vi "Read RequestMessage.vi"(8 "error in (no error)":errorcluster, 11 "HttpResponseMessage in":refnum<class "HttpResponseMessage.lvclass">) -> (0 "error out":errorcluster, 2 "HttpRequestMessage out":refnum<class "HttpRequestMessage.lvclass">, 3 "HttpResponseMessage out":refnum<class "HttpResponseMessage.lvclass">)   [LabVIEW 2018, in "LabVIEWHTTPClient_NET.lvlib" / "HttpResponseMessage.lvclass"]
uses:
  HttpResponseMessage.lvclass
  HttpRequestMessage/HttpRequestMessage.lvclass
  HttpResponseMessage.lvclass/HttpResponseMessage.ctl
  System.Net.Http
  Accessors/Write HttpRequestMessage.vi
  Accessors/Read NET_HttpReponseMessage.vi
  Accessors/Read HttpRequestMessage.vi
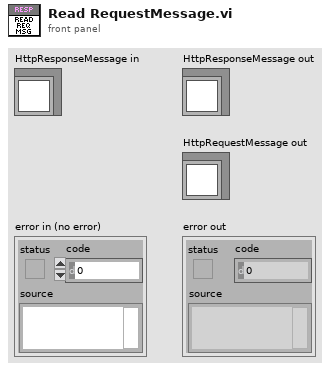
[diagram p1: front panel]
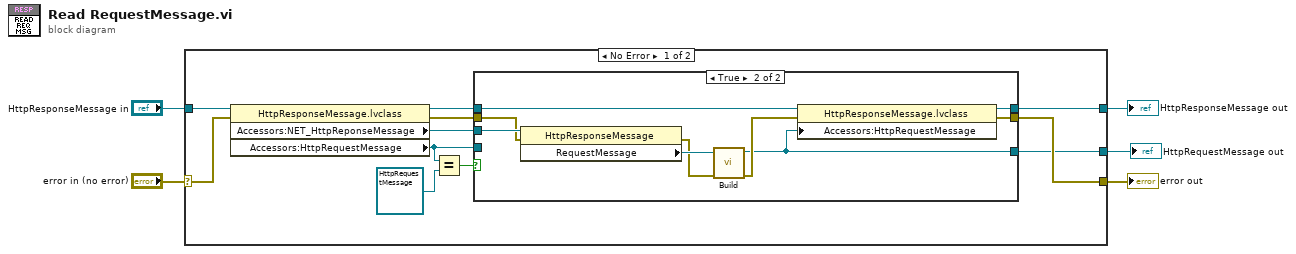
[diagram p0: block diagram]
diagram:
  n1 = case shown="No Error" "error in (no error)" {
    selector: "error in (no error)" -> [w16 w30]
    tunnel: [w11 w30] -> w4
    tunnel: [w9 w29] -> w2
    tunnel: "HttpResponseMessage in" -> [w15 w29]
    tunnel: [w8 _] -> w1
    frame No Error {
      n2 = property class="HttpResponseMessage.lvclass"(reference=w15, error in=w16) -> (reference out=w10:refnum<class "HttpResponseMessage.lvclass">, error out=w13:errorcluster, "Accessors:NET_HttpReponseMessage"=w14:refnum<k24>, "Accessors:HttpRequestMessage"=w6:refnum<class "HttpRequestMessage.lvclass">)
      n3 = Equal?(x=w6, y=refnum<class "HttpRequestMessage.lvclass"> refnum) -> (x = y?=w7:bool)
      n4 = case shown="True" w7 {
        tunnel: w14 -> [_ w28]
        tunnel: w13 -> [w18 w24]
        tunnel: [w18 w23] -> w11
        tunnel: w10 -> [w19 w22]
        tunnel: [w19 w21] -> w9
        tunnel: [w17 w20] -> w8
        tunnel: w6 -> [w17 _]
        frame False {
        }
        frame True {
          n5 = property class="HttpResponseMessage"(reference=w28, error in=w24) -> (error out=w26:errorcluster, "RequestMessage"=w27:refnum<k24>)  [unwired: 1 out]
          n6 = call "Build.vi"("error in (no error)"=w26, "HttpRequestMessage"=w27) -> ("error out"=w25:errorcluster, "HttpRequestMessage out"=w20:refnum<class "HttpRequestMessage.lvclass">)  [unwired: 8 in]
          n7 = property class="HttpResponseMessage.lvclass"(reference=w22, error in=w25, "Accessors:HttpRequestMessage"=w20) -> (reference out=w21:refnum<class "HttpResponseMessage.lvclass">, error out=w23:errorcluster)
        }
      }
    }
    frame Error {
    }
  }
  "error out" <- w4
  "HttpResponseMessage out" <- w2
  "HttpRequestMessage out" <- w1
